vi "Get_Port_status.vi"(8 "error in (no error)":errorcluster, 10 "CH":i32, 11 "Cypress in":refnum<class "Cypress.lvclass">) -> (0 "error out":errorcluster, 1 "Expected Response":string, 2 "Command to Send":string, 3 "Cypress out":refnum<class "Cypress.lvclass">)   [LabVIEW 2020, in "Cypress.lvclass"]
uses:
  Cypress.lvclass
  Abstract/Serial Device/Combo Box Comandos.ctl
  Abstract/Serial Device/Combo Box Devices.ctl
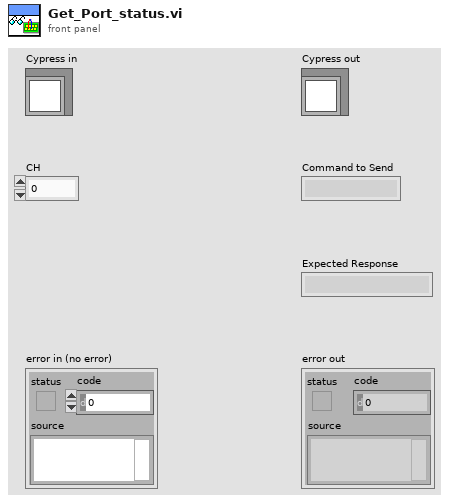
[diagram p1: front panel]
types:
  T1 = typedef "Combo Box Devices.ctl" = string
  T2 = typedef "Combo Box Comandos.ctl" = string
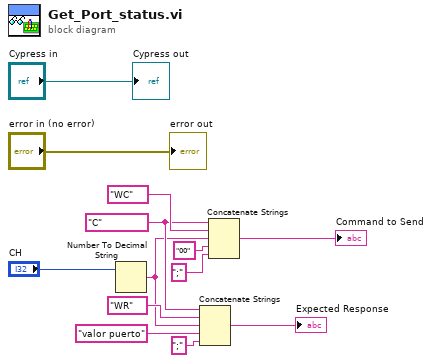
[diagram p0: block diagram]
diagram:
  w10 = T1 "C" ("Serial Devide Brand")
  n1 = Number To Decimal String(number="CH") -> (decimal integer string=w8:string)  [unwired: 1 in]
  n2 = Concatenate Strings(w10, T2 "WR" ("Respuesta"), w8, "valor puerto" ("string"), ";" ("string")) -> (→"Expected Response":string)
  n3 = Concatenate Strings(w10, T2 "WC" ("Command"), w8, "00" ("string"), ";" ("string")) -> (→"Command to Send":string)
  "error out" <- "error in (no error)"
  "Cypress out" <- "Cypress in"
